vi "FITS_OpenFile.vi"(7 "mode":i32(ring) items=["READ ONLY", "READ/WRITE"], 8 "error in":errorcluster, 10 "filename":string) -> (0 "error out":errorcluster, 2 "result":i32, 3 "fp out":u64)   [LabVIEW 2016]
panel:
  in  "fp in":u64
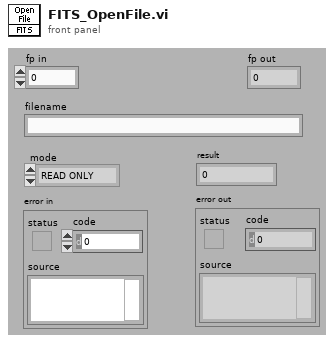
[diagram p1: front panel]
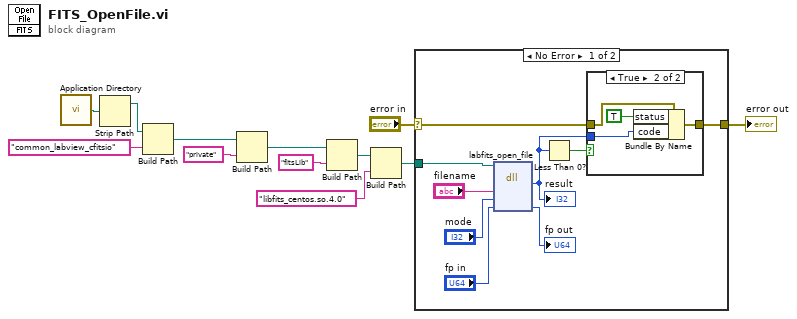
[diagram p0: block diagram]
diagram:
  n1 = call <vilib>:"Application Directory.vi"() -> ("Application Directory"=w4:path)
  n2 = Strip Path(path=w4) -> (stripped path=w3:path)  [unwired: 1 out]
  n3 = Build Path(base path=w3, name or relative path="common_labview_cfitsio") -> (appended path=w9:path)
  n4 = Build Path(base path=w9, name or relative path="private") -> (appended path=w7:path)
  n5 = Build Path(base path=w7, name or relative path="fitsLib") -> (appended path=w5:path)
  n6 = Build Path(base path=w5, name or relative path="libfits_centos.so.4.0") -> (appended path=w1:path)
  n7 = case shown="No Error" "error in" {
    selector: "error in" -> [w19 w27]
    tunnel: [w18 w27] -> w11
    tunnel: w1 -> [w13 _]
    frame No Error {
      n8 = dll-call lib="usr/local/lib/libfits.so" fn="labfits_open_file"(path in=w13, "filename"="filename", "mode"="mode", "fp"="fp in") -> ("return type"=w17:i32, "fp"=→"fp out":u64)  [unwired: 4 in, 2 out]
      "result" <- w17
      n9 = Less Than 0?(x=w17) -> (x < 0?=w20:bool)
      n10 = case shown="True" w20 {
        tunnel: w19 -> [w22 w24]
        tunnel: [w22 w23] -> w18
        tunnel: w17 -> [_ w25]
        frame False {
        }
        frame True {
          n11 = Bundle By Name(cluster=w24, "status"=TRUE, "code"=w25) -> (w23:errorcluster)
        }
      }
    }
    frame Error {
    }
  }
  "error out" <- w11
